vi "Wait for Connection.vi"(8 "error in (no error)":errorcluster, 11 "timeout ms (wait forever: -1)":i32) -> (0 "error out":errorcluster, 3 "connection ID":refnum<k5>)   [LabVIEW 2017, in "DSF Core.lvlib" / "Data Server Thread.lvclass"]
uses:
  Data Server Thread.lvclass
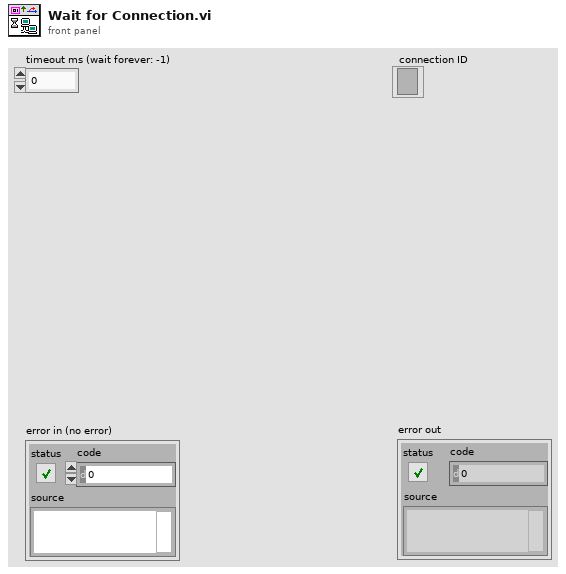
[diagram p1: front panel]
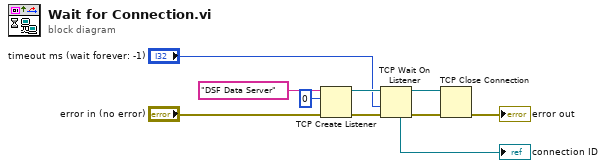
[diagram p0: block diagram]
diagram:
  n1 = TCP Create Listener(8:"error in (no error)", 10:u16 0 ("port"), 11:"DSF Data Server" ("service name")) -> (0:w9:errorcluster, 3:w10:refnum<k5>)  [unwired: 2 in, 1 out]
  n2 = TCP Wait On Listener(8:w9, 9:"timeout ms (wait forever: -1)", 11:w10) -> (0:w3:errorcluster, 3:w2:refnum<k5>, 4:→"connection ID":refnum<k5>)  [unwired: 1 in, 2 out]
  n3 = TCP Close Connection(connection ID=w2, error in (no error)=w3) -> (error out=→"error out":errorcluster)  [unwired: 1 in, 1 out]
